vi "Open Safety Relay.vi"(8 "error in (no error)":errorcluster, 11 "DeepU Test Stand in":refnum<class "DeepU Test Stand.lvclass">) -> (0 "error out":errorcluster, 3 "DeepU Test Stand out":refnum<class "DeepU Test Stand.lvclass">)   [LabVIEW 2019, in "Test Stands.lvlib" / "DeepU Test Stand.lvclass"]
uses:
  DeepU Test Stand.lvclass
  DeepU Test Stand.lvclass/DeepU Test Stand.ctl
  <vilib>/DAQmx/write.llb/DAQmx Write (Digital Bool 1Line 1Point).vi
  <vilib>/DAQmx/miscellaneous.llb/DAQmx Fill In Error Info.vi
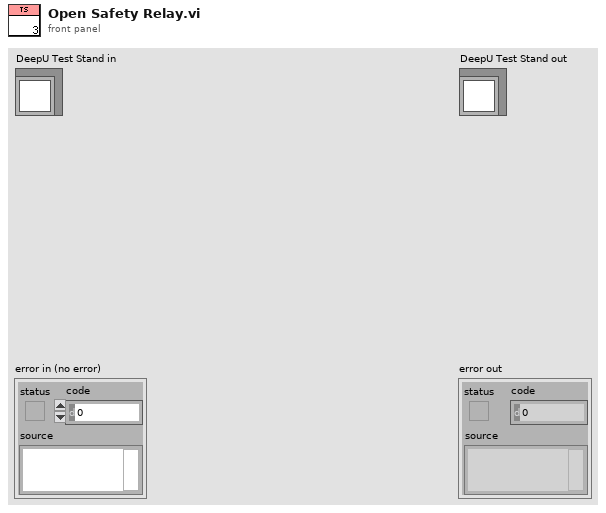
[diagram p1: front panel]
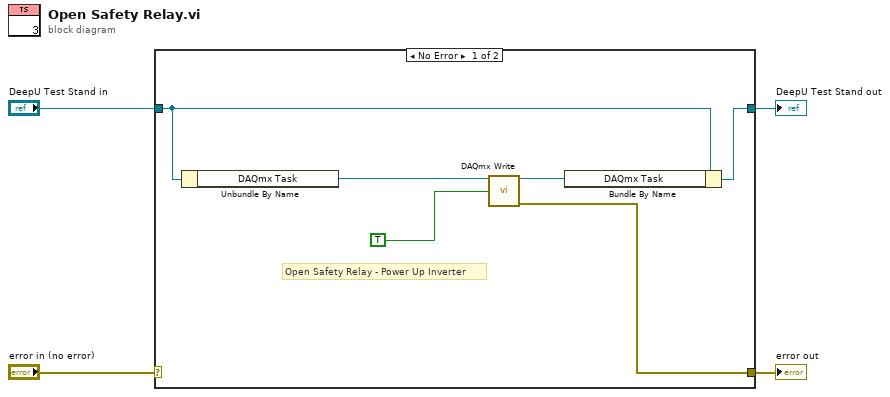
[diagram p0: block diagram]
diagram:
  n1 = case shown="No Error" "error in (no error)" {
    selector: "error in (no error)" -> [_ w12]
    tunnel: [w6 w12] -> w3
    tunnel: [w7 w11] -> w1
    tunnel: "DeepU Test Stand in" -> [w9 w11]
    frame No Error {
      # "Open Safety Relay - Power Up Inverter"
      n2 = Unbundle By Name(w9) -> ("DAQmx Task"=w10:refnum<k21>)
      n3 = call-poly <vilib>:"DAQmx Write.vi"("task/channels in"=w10, "data"=TRUE) -> ("task out"=w8:refnum<k21>, "error out"=w6:errorcluster)  [unwired: 11 in, 1 out]
      n4 = Bundle By Name(cluster=w9, "DAQmx Task"=w8) -> (w7:refnum<class "DeepU Test Stand.lvclass">)
    }
    frame Error {
    }
  }
  "error out" <- w3
  "DeepU Test Stand out" <- w1
